vi "Main.vi"() -> ()   [LabVIEW 2014]
doc: "Use this template to build a simple state machine design pattern. Each state executes code and determines which state to transition to."
uses:
  controls/Data1.ctl
  controls/Payjson.ctl
  controls/State.ctl
panel:
  in  "PrintNum":u16 caption="列印數:"
  in  "ReScanNG":i32
  in  "InputBarCode":string
  in  "Exit":bool
  in  "Data":T1
  # "This template is for the Simple State Machine design pattern.\n\nSee the block diagram for more information on how to use this template."
  # "These controls have associated \"Value Changed\" events configured in the Event Structure on the diagram.\n\nReplace them (and reconfigure the Event Structure) with the controls you need for your application."
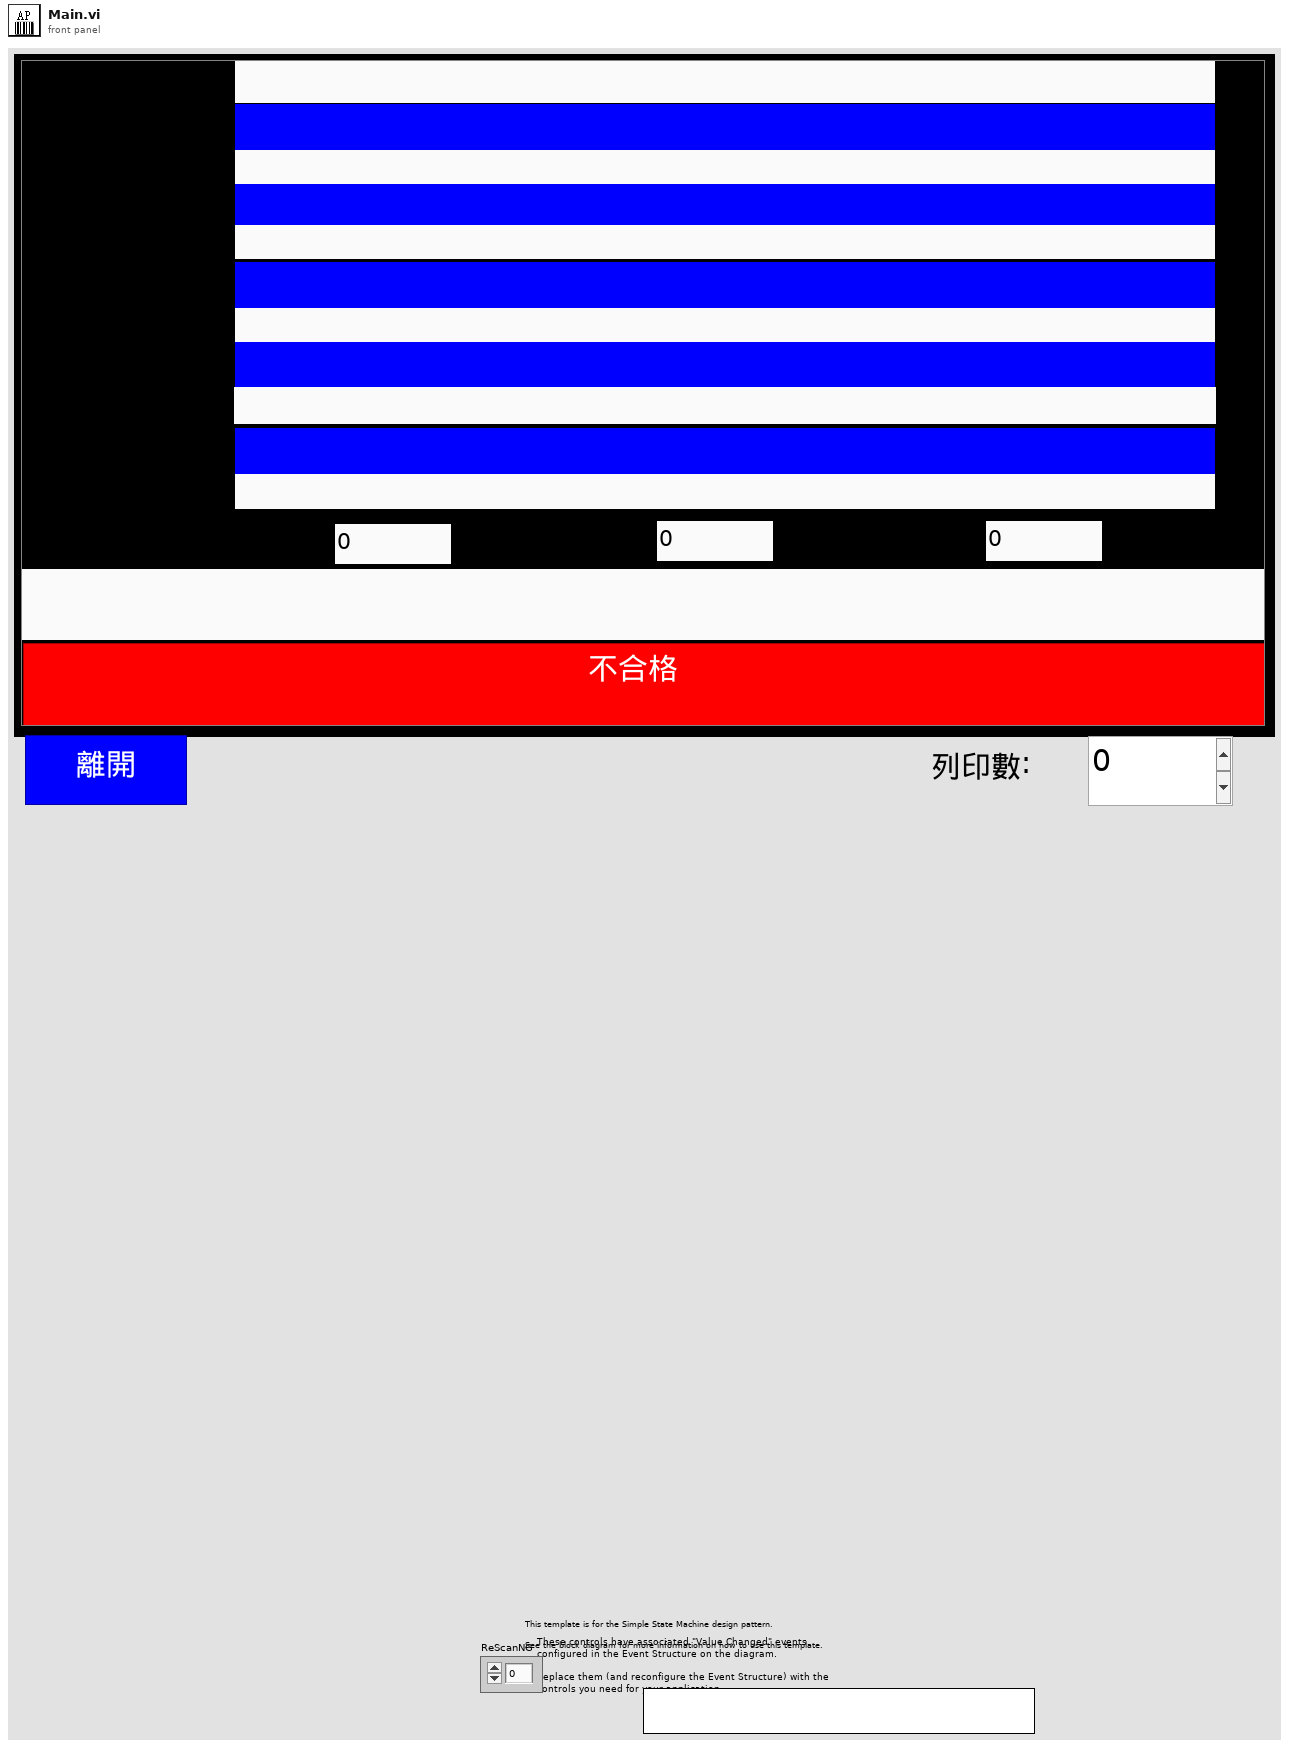
[diagram p1: front panel]
types:
  T1 = typedef "Data1.ctl" = cluster{"Date":string, "BarCode1":string, "BarCode2":string, "BarCode3":string, "Message":string, "OK Count":u16, "NG Count":u16, "Total Count":u16, "ModelData":string[][], "OK&NG":bool, "COM1":refnum<visa-resource-name>, "COM2":refnum<visa-resource-name>, "IO":i32, "Time":u32, "TCP":refnum<k5>, "TCP 2":refnum<k5>, "COM1 2":refnum<visa-resource-name>, "CheckNum":string, "BarCode1_1":string, "BarCode2_1":string, "BarCode3_1":string, "日期":string, "機種":string, "機號":string, "商品條碼1":string, "OK_1":string, "OK":string, "NG":string, "NG_1":string, "Total":string, "Total_1":string, "ClaerTime":u32, "Pjson":T2, "LotNo":string[], "CheckParsArray":string[], "BarCode4":string, "BarCode4_1":string, "商品條碼2":string, "BarCode5":string, "BarCode5_1":string, "商品條碼3":string, "ReScanNG":i32, "NGTimeCT":u32}
  T2 = typedef "Payjson.ctl" = cluster{"DEPT":string, "LINE":string, "STANO":string, "WORKNO":string, "PRODSN":string, "COMPNTID":string, "COMPNTLOT":string, "COMPNTSN":string, "USEDQTY":i16, "OPDATE":string, "OPUSER":string, "RECVDATE":string, "MMODU":string}[]
  T3 = typedef "State.ctl" = enum16{"int", "Initalize0", "Initialize", "Wait for Scan", "State 1", "State 2", "NG", "NG1", "OK", "OKNG", "OKNG1", "Exit"}
  T4 = enum8{"Enabled", "Disabled", "Disabled and Grayed Out"}
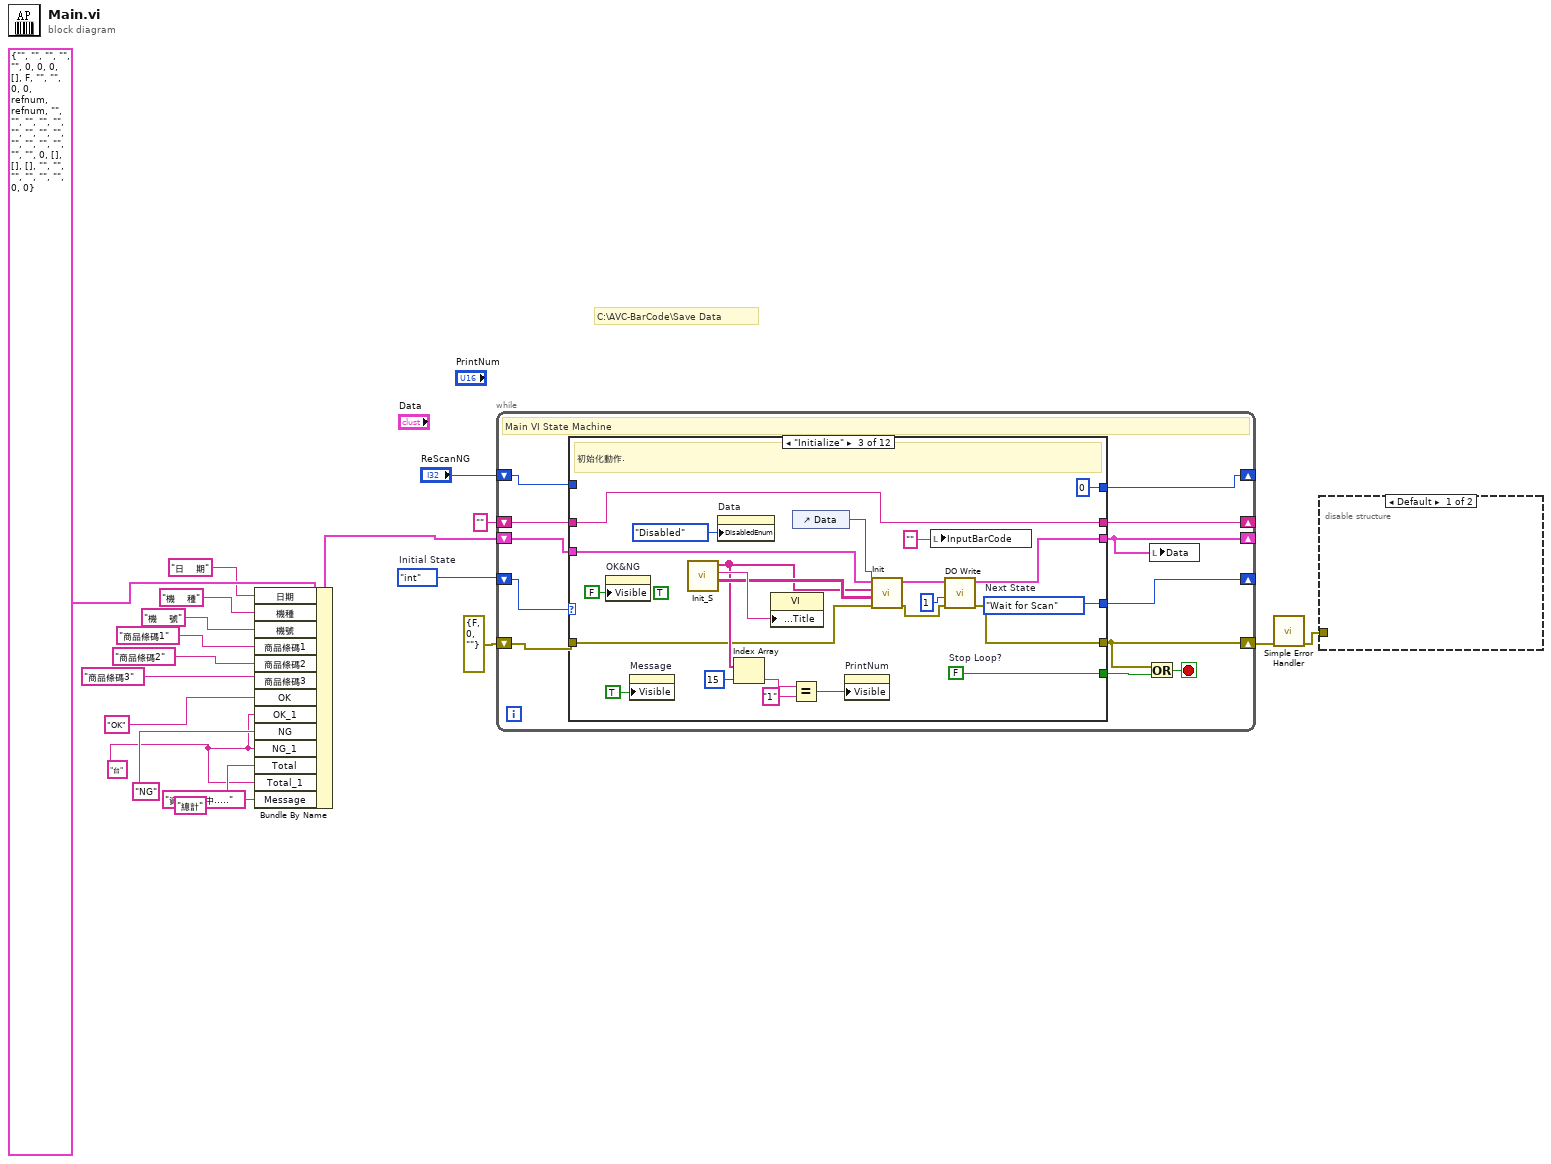
[diagram p0: block diagram]
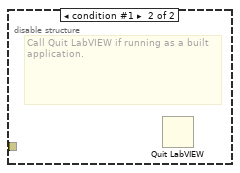
[diagram p2: hidden frame]
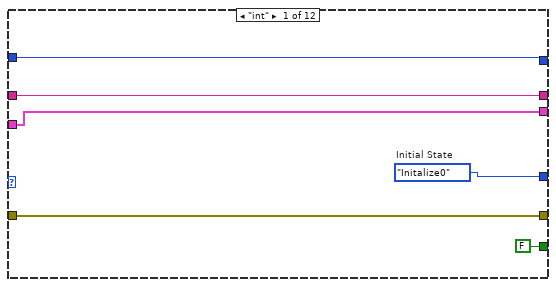
[diagram p3: hidden frame]
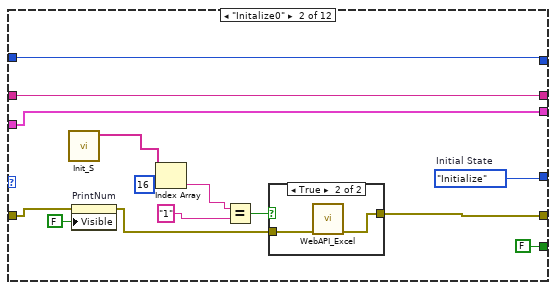
[diagram p4: hidden frame]
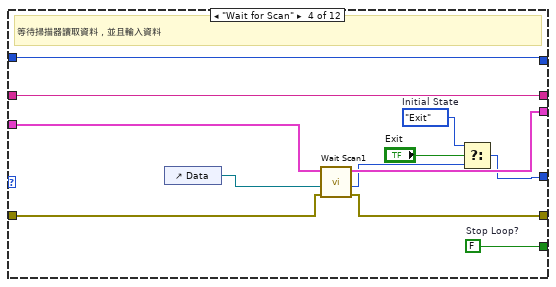
[diagram p6: hidden frame]
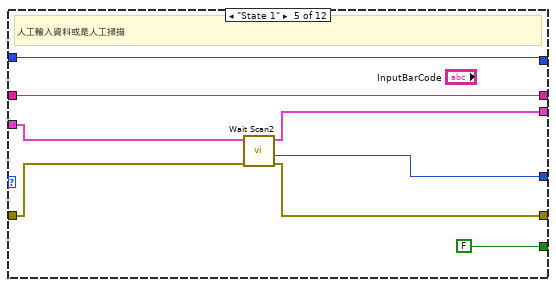
[diagram p7: hidden frame]
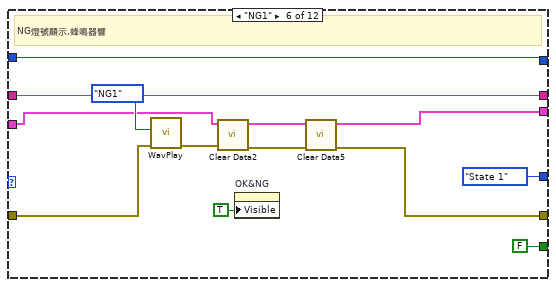
[diagram p8: hidden frame]
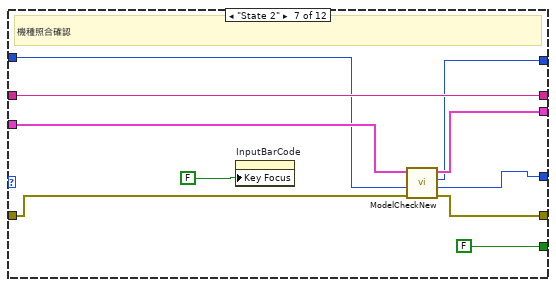
[diagram p9: hidden frame]
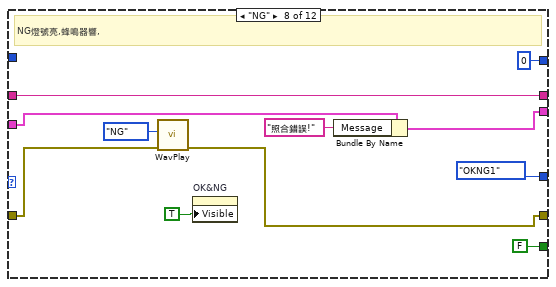
[diagram p10: hidden frame]
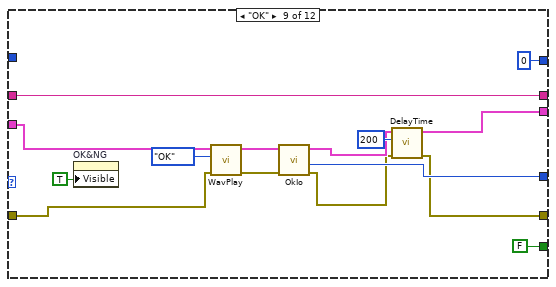
[diagram p11: hidden frame]
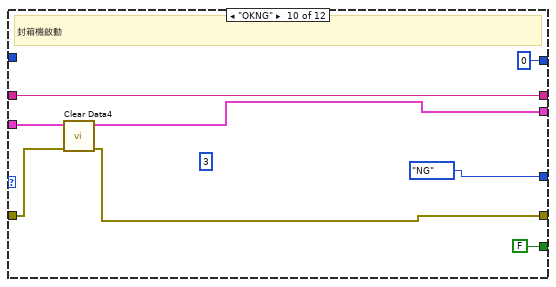
[diagram p12: hidden frame]
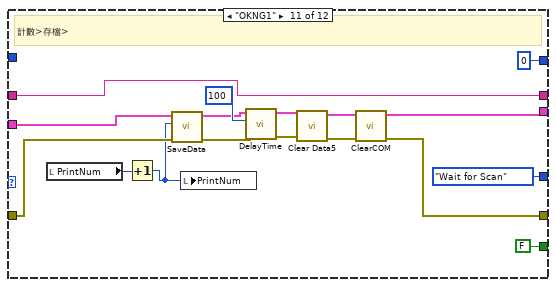
[diagram p13: hidden frame]
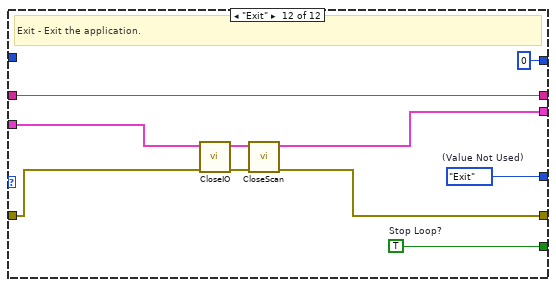
[diagram p14: hidden frame]
diagram:
  w5 = "台" ("OK_1")
  w16 = State."int"  # Initial State
  # "C:\\AVC-BarCode\\Save Data"
  n1 = Bundle By Name(cluster=T1 {"Date"="", "BarCode1"="", "BarCode2"="", "BarCode3"="", "Message"="", "OK Count"=0, "NG Count"=0, "Total Count"=0, "ModelData"=[], "OK&NG"=FALSE, "COM1"="", "COM2"="", "IO"=0, "Time"=0, "TCP"=refnum, "TCP 2"=refnum, "COM1 2"="", "CheckNum"="", "BarCode1_1"="", "BarCode2_1"="", "BarCode3_1"="", "日期"="", "機種"="", "機號"="", "商品條碼1"="", "OK_1"="", "OK"="", "NG"="", "NG_1"="", "Total"="", "Total_1"="", "ClaerTime"=0, "Pjson"=[], "LotNo"=[], "CheckParsArray"=[], "BarCode4"="", "BarCode4_1"="", "商品條碼2"="", "BarCode5"="", "BarCode5_1"="", "商品條碼3"="", "ReScanNG"=0, "NGTimeCT"=0} ("Data"), "日期"="日    期", "機種"="機    種", "機號"="機    號" ("機種"), "商品條碼1"="商品條碼1" ("機種"), "商品條碼2"="商品條碼2", "商品條碼3"="商品條碼3", "OK"="OK", "OK_1"=w5, "NG"="NG", "NG_1"=w5, "Total"="總計", "Total_1"=w5, "Message"="資料下載中.....") -> (w12:T1)
  n2 = while {
    shift-right: [w29] -> _
    shift-left: w16 -> [w27]
    shift-right: [w20] -> _
    shift-left: w12 -> [w25]
    shift-right: [w26] -> w18
    shift-left: errorcluster {"status"=FALSE, "code"=0, "source"=""} ("error constant") -> [w28]
    shift-right: [w24] -> _
    shift-left: "" ("InputBarCode") -> [w23]
    shift-right: [w22] -> _
    shift-left: "ReScanNG" -> [w21]
    stop <- w30 stop-if-true
    # "Main VI State Machine"
    n3 = case shown="\"Initialize\"" w27 {
      tunnel: [FALSE ("Stop Loop?") FALSE ("Stop Loop?") w77 w89 FALSE ("Stop Loop?") FALSE ("Stop Loop?") FALSE ("Stop Loop?") FALSE ("Stop Loop?") FALSE ("Stop Loop?") FALSE ("Stop Loop?") FALSE ("Stop Loop?") w180] -> w31
      tunnel: w28 -> [w37 w48 w55 w83 w92 w105 w117 w126 w134 w150 w169 w172]
      tunnel: [w37 w45 w71 w82 w91 w100 w116 w122 w136 w147 w156 w177] -> w26
      tunnel: w25 -> [w32 w49 w63 w88 w94 w103 w119 w124 w144 w149 w170 w173]
      tunnel: [w32 w49 w73 w87 w93 w99 w118 w123 w138 w148 w157 w178] -> w20
      tunnel: [w36 w46 w76 w81 w90 State."State 1" ("(Value Not Used)") w115 State."OKNG1" ("(Value Not Used)") w142 State."NG" ("(Value Not Used)") State."Wait for Scan" ("(Value Not Used)") w179] -> w29
      tunnel: [w33 w50 w68 w79 w95 w108 w114 w130 w141 w152 w164 w176] -> w24
      tunnel: w23 -> [w33 w50 w68 w79 w95 w108 w114 w130 w141 w152 w164 w176]
      tunnel: [w34 w51 0 ("ReScanNG") w78 w96 w107 w111 0 ("ReScanNG") 0 ("ReScanNG") 0 ("ReScanNG") 0 ("ReScanNG") 0 ("ReScanNG")] -> w22
      tunnel: w21 -> [w34 w51 _ w78 w96 w107 w112 _ _ _ _ _]
      frame "int" {
        w36 = State."Initalize0"  # Initial State
      }
      frame "Initalize0" {
        w46 = State."Initialize"  # Initial State
        n4 = call "Init_S.vi"() -> ("Path_out"=w42:string[])  [unwired: 9 in, 2 out]
        n5 = property on="PrintNum" class="DigNum (strict)"(error in=w48, "Visible"=FALSE) -> (error out=w47:errorcluster)  [unwired: 1 in, 1 out]
        n6 = Index Array(array=w42, index=16) -> (element=w40:string)
        n7 = Equal?(x=w40, y="1") -> (x = y?=w38:bool)
        n8 = case shown="True" w38 {
          tunnel: w47 -> [w52 w54]
          tunnel: [w52 w53] -> w45
          frame False {
          }
          frame True {
            n9 = call "WebAPI_Excel.vi"("error in (no error)"=w54) -> ("error out"=w53:errorcluster)  [unwired: 10 in]
          }
        }
      }
      frame "Initialize" {
        (unwired) TRUE ("Key Focus")
        w77 = FALSE  # Stop Loop?
        w76 = State."Wait for Scan"  # Next State
        # "初始化動作."
        n10 = property on="OK&NG" class="Bool (strict)"("Visible"=FALSE) -> ()  [unwired: 2 in, 2 out]
        n11 = property on="Message" class="Str"("Visible"=TRUE) -> ()  [unwired: 2 in, 2 out]
        n12 = call "Init_S.vi"() -> ("All_info"=w62:string[][], "Title"=w65:string, "Path_out"=w57:string[])  [unwired: 9 in]
        n13 = property on="Data" class="Clust (strict)"("DisabledEnum"=T4."Disabled" ("Disabled")) -> ()  [unwired: 2 in, 2 out]
        n14 = Index Array(array=w57, index=15) -> (element=w59:string)
        n15 = property class="VI"("Front Panel.Title"=w65) -> ()  [unwired: 2 in, 2 out]
        n16 = Equal?(x=w59, y="1") -> (x = y?=w56:bool)
        n17 = control-ref of="Data"() -> (w61:refnum<vi>)
        n18 = property on="PrintNum" class="DigNum (strict)"("Visible"=w56) -> ()  [unwired: 2 in, 2 out]
        n19 = call "Init.vi"("Clust Refnum"=w61, "error in (no error)"=w55, "All_info"=w62, "Path_out"=w57, "Data"=w63) -> ("error out"=w72:errorcluster, "Data Out"=w74:T1)  [unwired: 5 in]
        n20 = local write "InputBarCode"("") -> ()
        n21 = call "DO Write.vi"("error in (no error)"=w72, "data"=u8 1, "Data In"=w74) -> ("error out"=w71:errorcluster, "Data Out"=w73:T1)  [unwired: 7 in]
      }
      frame "Wait for Scan" {
        w85 = State."Exit"  # Initial State
        w89 = FALSE  # Stop Loop?
        # "等待掃描器讀取資料，並且輸入資料"
        n22 = control-ref of="Data"() -> (w80:refnum<vi>)
        n23 = call "Wait Scan1.vi"("error in (no error)"=w83, "Clust Refnum"=w80, "Data In"=w88) -> ("error out"=w82:errorcluster, "States"=w84:T3, "Data Out"=w87:T1)  [unwired: 6 in]
        n24 = Select(t=w85, s="Exit", f=w84) -> (s? t:f=w81:T3)
      }
      frame "State 1" {
        # "人工輸入資料或是人工掃描"
        n25 = call "Wait Scan2.vi"("error in (no error)"=w92, "Data In"=w94) -> ("error out"=w91:errorcluster, "States"=w90:T3, "Data Out"=w93:T1)  [unwired: 7 in]
      }
      frame "NG1" {
        # "NG燈號顯示,蜂鳴器響"
        n26 = call "WavPlay.vi"("error in (no error)"=w105, "OkNg"=enum16{"OK", "NG", "NG1", "SCAN"}."NG1") -> ("error out"=w104:errorcluster)  [unwired: 9 in]
        n27 = call "Clear Data2.vi"("error in (no error)"=w104, "Data In"=w103) -> ("error out"=w102:errorcluster, "Data out"=w101:T1)  [unwired: 8 in]
        n28 = property on="OK&NG" class="Bool (strict)"("Visible"=TRUE) -> ()  [unwired: 2 in, 2 out]
        n29 = call "Clear Data5.vi"("error in (no error)"=w102, "Data In"=w101) -> ("error out"=w100:errorcluster, "Data out"=w99:T1)  [unwired: 8 in]
      }
      frame "State 2" {
        # "機種照合確認"
        n30 = property on="InputBarCode" class="Str"("Key Focus"=FALSE) -> ()  [unwired: 2 in, 2 out]
        n31 = call "ModelCheckNew.vi"("error in (no error)"=w117, "ReScanNG"=w112, "Data In"=w119) -> ("error out"=w116:errorcluster, "States"=w115:T3, "ReScanNG"=w111:i32, "Data Out"=w118:T1)  [unwired: 5 in]
      }
      frame "NG" {
        # "NG燈號亮,蜂鳴器響,"
        n32 = call "WavPlay.vi"("error in (no error)"=w126, "OkNg"=enum16{"OK", "NG", "NG1", "SCAN"}."NG") -> ("error out"=w122:errorcluster)  [unwired: 9 in]
        n33 = property on="OK&NG" class="Bool (strict)"("Visible"=TRUE) -> ()  [unwired: 2 in, 2 out]
        n34 = Bundle By Name(cluster=w124, "Message"="照合錯誤!") -> (w123:T1)
      }
      frame "OK" {
        n35 = property on="OK&NG" class="Bool (strict)"("Visible"=TRUE) -> ()  [unwired: 2 in, 2 out]
        n36 = call "WavPlay.vi"("error in (no error)"=w134, "OkNg"=enum16{"OK", "NG", "NG1", "SCAN"}."OK") -> ("error out"=w133:errorcluster)  [unwired: 9 in]
        n37 = call "OkIo.vi"("error in (no error)"=w133, "Data In"=w144) -> ("error out"=w137:errorcluster, "States"=w142:T3, "Data Out"=w139:T1)  [unwired: 7 in]
        n38 = call "DelayTime.vi"("error in (no error)"=w137, "Time"=u32 200, "Data In"=w139) -> ("error out"=w136:errorcluster, "Data Out"=w138:T1)  [unwired: 7 in]
      }
      frame "OKNG" {
        (unwired) 3 ("index")
        # "封箱機啟動"
        n39 = call "Clear Data4.vi"("error in (no error)"=w150, "Data In"=w149) -> ("error out"=w147:errorcluster, "Data out"=w148:T1)  [unwired: 8 in]
      }
      frame "OKNG1" {
        # "計數>存檔>"
        n40 = local read "PrintNum"() -> (w155:u16)
        n41 = Increment(x=w155) -> (x+1=w154:u16)
        n42 = call "SaveData.vi"("error in (no error)"=w169, "PrintNum"=w154, "Data In"=w170) -> ("error out"=w166:errorcluster, "Data Out"=w167:T1)  [unwired: 7 in]
        n43 = local write "PrintNum"(w154) -> ()
        n44 = call "DelayTime.vi"("error in (no error)"=w166, "Time"=u32 100, "Data In"=w167) -> ("error out"=w160:errorcluster, "Data Out"=w161:T1)  [unwired: 7 in]
        n45 = call "Clear Data5.vi"("error in (no error)"=w160, "Data In"=w161) -> ("error out"=w158:errorcluster, "Data out"=w159:T1)  [unwired: 8 in]
        n46 = call "ClearCOM.vi"("error in (no error)"=w158, "Data In"=w159) -> ("error out"=w156:errorcluster, "Data out"=w157:T1)  [unwired: 8 in]
      }
      frame "Exit" {
        w180 = TRUE  # Stop Loop?
        w179 = State."Exit"  # (Value Not Used)
        # "Exit - Exit the application."
        n47 = call "CloseIO.vi"("error in (no error)"=w172, "Data In"=w173) -> ("error out"=w174:errorcluster, "Data Out"=w175:T1)  [unwired: 8 in]
        n48 = call "CloseScan.vi"("error in (no error)"=w174, "Data In"=w175) -> ("error out"=w177:errorcluster, "Data Out"=w178:T1)  [unwired: 8 in]
      }
    }
    n49 = Or(x=w26, y=w31) -> (x .or. y?=w30:bool)
    n50 = local write "Data"(w20) -> ()
  }
  n51 = call <vilib>:"Simple Error Handler.vi"("error in (no error)"=w18) -> ("error out"=w17:errorcluster)  [unwired: 4 in, 4 out]
  n52 = disable-structure shown="Default" {
    disable-tunnel: w17 -> [_ _]
    frame condition #0 (active) {
    }
    frame condition #1 {
      # "Call Quit LabVIEW if running as a built application."
      n53 = Quit LabVIEW() -> ()  [unwired: 1 in]
    }
  }
